vi "jettl.vi"(0 "Path":path, 4 "Creator":refnum<user-event>, 6 "Creator Alias":string, 8 "Self Alias":string, 9 "Queue of Init":refnum<queue>, 10 "Actor":refnum<class "Actor.lvclass">) -> ()   [LabVIEW 2021, in "jettl.lvlib" / "Temporary Actor.lvlib" / "jettl Actor.lvclass"]
uses:
  jettl Actor.lvclass
  Actor/Actor.lvclass
  Msg/Msg.lvclass
  Init.ctl
  C:/git/jettl/jettl/jettl/Actor/Actor.lvclass
  jettl Actor.lvclass/jettl Actor.ctl
  Addresses Strategy/Addresses Strategy.lvlib
  Last Ack Msg/Last Ack Msg.lvlib
  C:/git/jettl/jettl/jettl/Temporary Actor/Actor/Actor.lvclass
  C:/git/jettl/jettl/jettl/Last Ack Msg/Last Ack/Last Ack.lvclass
  C:/git/jettl/jettl/jettl/Setup Msg/Setup/Setup.lvclass
  C:/git/jettl/jettl/jettl/Teardown Msg/Teardown/Teardown.lvclass
  C:/git/jettl/jettl/jettl/Temporary Actor/jettl Actor/jettl Actor.lvclass
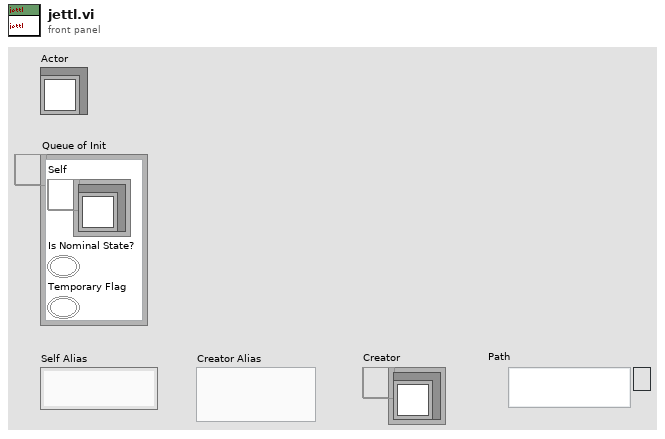
[diagram p1: front panel]
types:
  T1 = typedef "jettl.lvlib/Temporary Actor.lvlib/jettl Actor.lvclass/Init.ctl" = cluster{"Self":refnum<user-event>, "Is Nominal State?":bool, "Temporary Flag":bool}
  T2 = typedef "jettl.lvlib/Created Aliases.ctl" = set{string}
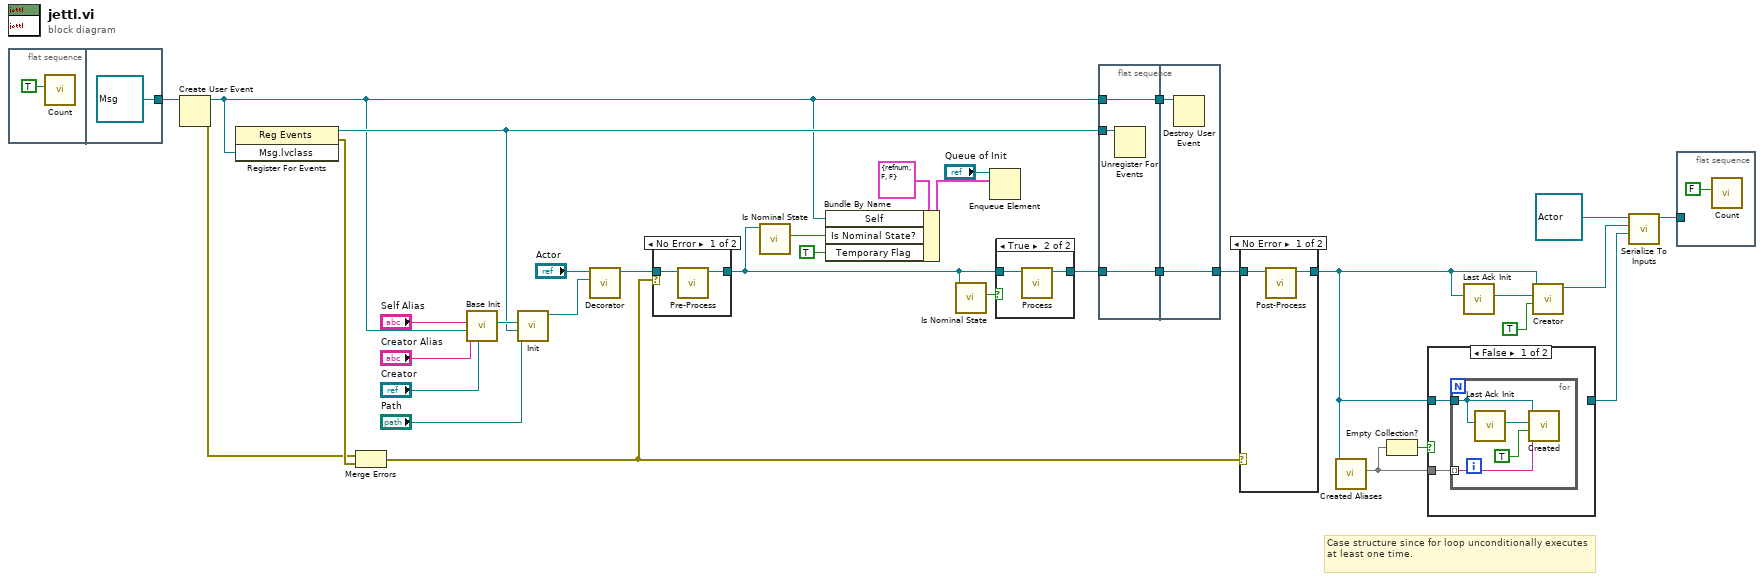
[diagram p0: block diagram]
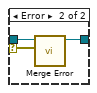
[diagram p2: hidden frame]
diagram:
  # "Case structure since for loop unconditionally executes at least one time."
  n1 = flat-sequence {
    tunnel: [refnum<class "Msg.lvclass"> refnum ("Msg.lvclass")] -> w28
    frame #0 {
      n2 = call "Count.vi"("Increment?"=TRUE) -> ()  [unwired: 11 in]
    }
    frame #1 {
    }
  }
  n3 = Create User Event(user event datatype=w28) -> (user event=w13:refnum<user-event>, error out=w30:errorcluster)  [unwired: 1 in]
  n4 = register-events(w13) -> (reference out=w20:refnum<event-registration>, error out=w32:errorcluster)  [unwired: 2 in]
  n5 = Merge Errors(w30, w32) -> (w17:errorcluster)
  n6 = call "Base Init.vi"("Creator"="Creator", "Creator Alias"="Creator Alias", "Self"=w13, "Self Alias"="Self Alias") -> ("Addresses Strategy out"=w29:refnum<class "Addresses Strategy.lvclass">)  [unwired: 7 in]
  n7 = call "Init.vi"("Path"="Path", "Register"=w20, "Addresses Strategy"=w29) -> ("jettl Actor out"=w26:refnum<class "jettl Actor.lvclass">)  [unwired: 8 in]
  n8 = call-dynamic "Decorator.vi"("Actor"=w26, "Actor in"="Actor") -> ("Actor out"=w25:refnum<class "Actor.lvclass">)  [unwired: 9 in]
  n9 = case shown="No Error" w17 {
    selector: w17 -> [_ w39]
    tunnel: [w38 w40] -> w24
    tunnel: w25 -> [w37 w41]
    frame No Error {
      n10 = call-dynamic "Pre-Process.vi"("Actor in"=w37) -> ("Actor out"=w38:refnum<class "Actor.lvclass">)  [unwired: 10 in]
    }
    frame Error {
      n11 = call-dynamic "Merge Error.vi"("Error"=w39, "Actor in"=w41) -> ("Actor out"=w40:refnum<class "Actor.lvclass">)  [unwired: 9 in]
    }
  }
  n12 = call-dynamic "Is Nominal State.vi"("Actor in"=w24) -> ("Is Nominal State?"=w12:bool)  [unwired: 10 in]
  n13 = Bundle By Name(cluster=T1 {"Self"=refnum, "Is Nominal State?"=FALSE, "Temporary Flag"=FALSE} ("element"), "Self"=w13, "Is Nominal State?"=w12, "Temporary Flag"=TRUE) -> (w14:T1)
  n14 = call-dynamic "Is Nominal State.vi"("Actor in"=w24) -> ("Is Nominal State?"=w10:bool)  [unwired: 10 in]
  n15 = Enqueue Element(queue="Queue of Init", element=w14) -> ()  [unwired: 2 in, 3 out]
  n16 = case shown="True" w10 {
    tunnel: w24 -> [w42 w44]
    tunnel: [w42 w43] -> w21
    frame False {
    }
    frame True {
      n17 = call-dynamic "Process.vi"("Actor in"=w44) -> ("Actor out"=w43:refnum<class "Actor.lvclass">)  [unwired: 10 in]
    }
  }
  n18 = flat-sequence {
    tunnel: [w47] -> w22
    tunnel: w21 -> [w47]
    tunnel: w20 -> [w46]
    tunnel: w13 -> [w45]
    tunnel: [w45] -> w19
    tunnel: [w49] -> w23
    tunnel: w22 -> [w49]
    tunnel: w19 -> [w48]
    frame #0 {
      n19 = Unregister For Events(event registration refnum=w46) -> ()  [unwired: 1 in, 1 out]
    }
    frame #1 {
      n20 = Destroy User Event(user event=w48) -> ()  [unwired: 1 in, 1 out]
    }
  }
  n21 = case shown="No Error" w17 {
    tunnel: w23 -> [w51 w52]
    tunnel: [w50 w52] -> w4
    frame No Error {
      n22 = call-dynamic "Post-Process.vi"("Actor in"=w51) -> ("Actor out"=w50:refnum<class "Actor.lvclass">)  [unwired: 10 in]
    }
    frame Error {
    }
  }
  n23 = call-dynamic "Created Aliases.vi"("Actor in"=w4) -> ("Created Aliases"=w6:T2)  [unwired: 10 in]
  n24 = Empty Collection?(1:w6) -> (0:w7:bool)
  n25 = case shown="False" w7 {
    tunnel: w6 -> [w54 _]
    tunnel: w4 -> [w53 w59]
    tunnel: [_ w59] -> w2
    frame False {
      n26 = for {
        tunnel: w53 -> [w56]
        tunnel: w54 -> [w58] mode=indexing
        n27 = call "Last Ack Init.vi"("Actor"=w56) -> ("Msg"=w55:refnum<class "Msg.lvclass">)  [unwired: 10 in]
        n28 = call-dynamic "Created.vi"("Created Alias"=w58, "Is Priority"=TRUE ("Priority?"), "Msg"=w55, "Actor in"=w56) -> ()  [unwired: 7 in, 1 out]
      }
    }
    frame True {
    }
  }
  n29 = call "Last Ack Init.vi"("Actor"=w4) -> ("Msg"=w8:refnum<class "Msg.lvclass">)  [unwired: 10 in]
  n30 = call-dynamic "Creator.vi"("Is Priority"=TRUE ("Priority?"), "Msg"=w8, "Actor in"=w4) -> ("Actor out"=w3:refnum<class "Actor.lvclass">)  [unwired: 8 in]
  n31 = call-dynamic "Serialize To Inputs.vi"("Input 2"=w2, "Input 1"=w3, "Actor in"=refnum<class "Actor.lvclass"> refnum ("jettl in")) -> ("Actor out"=w5:refnum<class "Actor.lvclass">)  [unwired: 8 in]
  n32 = flat-sequence {
    tunnel: w5 -> [_]
    frame #0 {
      n33 = call "Count.vi"("Increment?"=FALSE) -> ()  [unwired: 11 in]
    }
  }
